vi "ActDriveStraight.vi"(9 "FirstTime":bool, 10 "MaxSpeed (ft/s)":dbl, 11 "Dist (ft)":dbl) -> (0 "RightSpeedDemand":dbl, 1 "LeftSpeedDemand":dbl, 3 "Done":bool)   [LabVIEW 2020]
doc: "Robot will drive forward straight a set distance utilizing position control \n\nInputs:\n-- MaxSpeed -- Double -- in ft/s, the MaxSpeed the robot can go -- \n-- Dist (ft) -- Double -- Distance in feet you want the robot to go -- \n-- FirstTime -- Boolean -- Input true the first time this function is called, sets the target position -- \n\nOutputs:\n-- Done -- Bool -- has the robot reached its target distance\n-- LeftSpeedDemand -- Double -- Speed Demand for left drive train inorder to reach target -- \n-- RightSpeedDemand -- Double -- Speed Demand for left drive train inorder to reach target --"
uses:
  <vilib>/Rock Robotics/WPI/ThirdParty/JAS_Junk/TrajLib/Trajectory_Library.lvlib
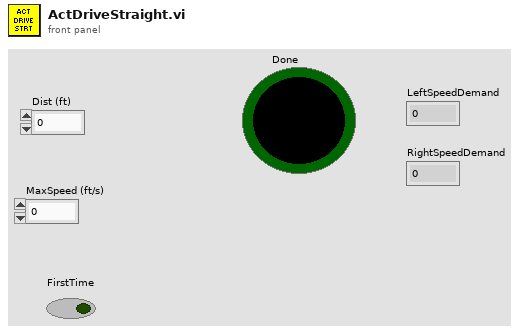
[diagram p1: front panel]
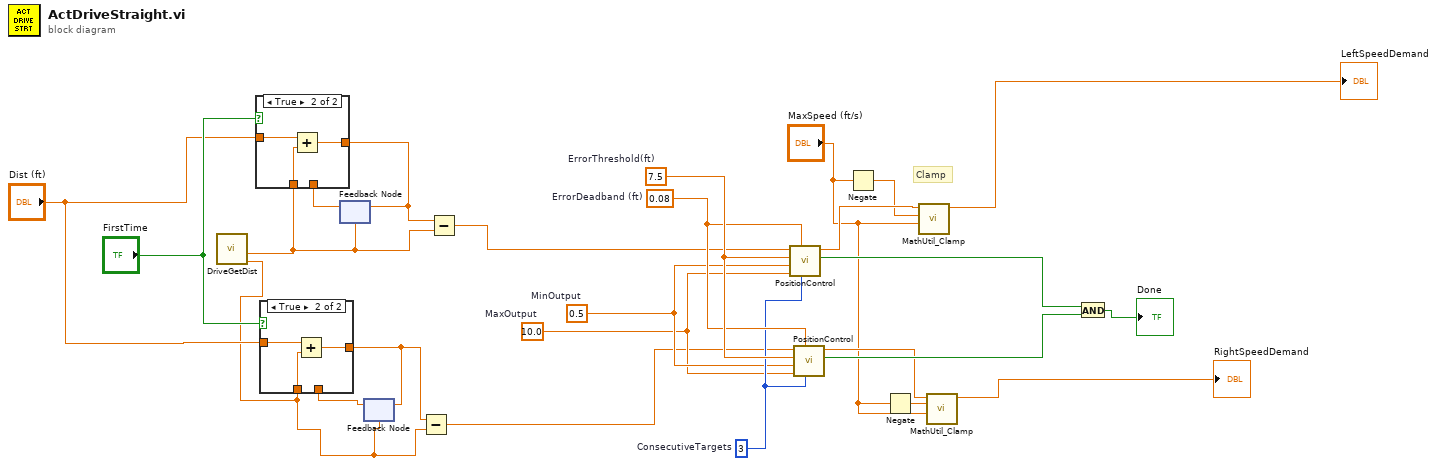
[diagram p0: block diagram]
diagram:
  w6 = 10.0  # MaxOutput
  w7 = 0.5  # MinOutput
  w17 = 3  # ConsecutiveTargets
  w20 = 0.08  # ErrorDeadband (ft)
  w21 = 7.5  # ErrorThreshold(ft)
  # "Clamp"
  n1 = call "DriveGetDist.vi"() -> ("Right dist"=w11:dbl, "Left dist"=w9:dbl)  [unwired: 10 in]
  n2 = feedback #1(w9) -> (w23:dbl)
  n3 = case shown="True" "FirstTime" {
    tunnel: "Dist (ft)" -> [_ w29]
    tunnel: w9 -> [_ w28]
    tunnel: [w26 w27] -> w10
    tunnel: w23 -> [w26 _]
    frame False {
    }
    frame True {
      n4 = Add(x=w29, y=w28) -> (x+y=w27:dbl)
    }
  }
  n5 = feedback-in #1(w10) -> ()
  n6 = feedback #2(w11) -> (w22:dbl)
  n7 = case shown="True" "FirstTime" {
    tunnel: "Dist (ft)" -> [_ w33]
    tunnel: w11 -> [_ w32]
    tunnel: [w30 w31] -> w3
    tunnel: w22 -> [w30 _]
    frame False {
    }
    frame True {
      n8 = Add(x=w33, y=w32) -> (x+y=w31:dbl)
    }
  }
  n9 = feedback-in #2(w3) -> ()
  n10 = Subtract(x=w3, y=w11) -> (x-y=w5:dbl)
  n11 = Subtract(x=w10, y=w9) -> (x-y=w4:dbl)
  n12 = call "PositionControl.vi"("ConsecutiveTargets"=w17, "ErrorDeadband"=w20, "MaxOutput"=w6, "MinOutput"=w7, "ErrorThreshold"=w21, "Error"=w4) -> ("OnTarget"=w18:bool, "OutputValue"=w16:dbl)  [unwired: 3 in, 1 out]
  n13 = call "PositionControl.vi"("ConsecutiveTargets"=w17, "ErrorDeadband"=w20, "MaxOutput"=w6, "MinOutput"=w7, "ErrorThreshold"=w21, "Error"=w5) -> ("OnTarget"=w19:bool, "OutputValue"=w14:dbl)  [unwired: 3 in, 1 out]
  n14 = Negate(x="MaxSpeed (ft/s)") -> (-x=w15:dbl)
  n15 = Negate(x="MaxSpeed (ft/s)") -> (-x=w13:dbl)
  n16 = call <vilib>:"MathUtil_Clamp.vi"("High Limit"="MaxSpeed (ft/s)", "Low Limit"=w15, "Value"=w16) -> ("Result"=→"LeftSpeedDemand":dbl)  [unwired: 8 in]
  n17 = call <vilib>:"MathUtil_Clamp.vi"("High Limit"="MaxSpeed (ft/s)", "Low Limit"=w13, "Value"=w14) -> ("Result"=→"RightSpeedDemand":dbl)  [unwired: 8 in]
  n18 = And(x=w18, y=w19) -> (x .and. y?=→"Done":bool)
